vi "Motor PWM.vi"() -> ()   [LabVIEW 2018]
panel:
  in  "Nome do canal":tag="C/PWM0"
  in  "stop":bool
  in  "PWM freq [Hz]":dbl(slide)=100.0 scale=40.0..40000.0
  in  "PWM duty  [%]":dbl(slide) scale=0.0..100.0
  in  "Iniciar o controle":bool
  # "CONTROLE DO MOTOR COM SINAL DE PWM"
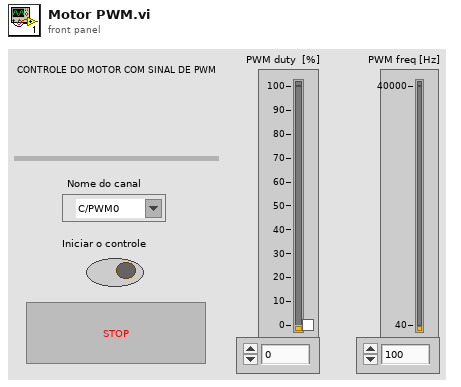
[diagram p1: front panel]
types:
  T1 = typedef "PWM.lvlib/PWM Reference.ctl" = cluster{"myRIO Reference":T2, "PWM Channels Enum":T6, "PWM Configuration":T7}
  T2 = typedef "myRIO Generic Hardware Reference.ctl" = cluster{"myRIO Model":T3, "myRIO Hardware Reference":T4}
  T3 = typedef "Hardware Version Enum.ctl" = enum16{"Unknown", "myRIO-1900", "myRIO-1950", "roboRIO", "NI ELVIS RIO CM"}
  T4 = typedef "myRIO v1.0 Reference.ctl" = cluster{"Generic FPGA Reference":T5, "Allow multiple opens":bool}
  T5 = typedef "Generic FPGA Reference.ctl" = refnum<k20>
  T6 = typedef "PWM Channels Enum.ctl" = enum16{"Not Connected", "C/PWM0", "C/PWM1", "A/PWM0", "A/PWM1", "A/PWM2", "B/PWM0", "B/PWM1", "B/PWM2", "PWM/PWM0", "PWM/PWM1", "PWM/PWM2", "PWM/PWM3", "PWM/PWM4", "PWM/PWM5", "PWM/PWM6", "PWM/PWM7", "PWM/PWM8", "PWM/PWM9"}
  T7 = typedef "PWM.lvlib/PWM Configuration.ctl" = cluster{"Frequency":dbl, "Duty Cycle":dbl}
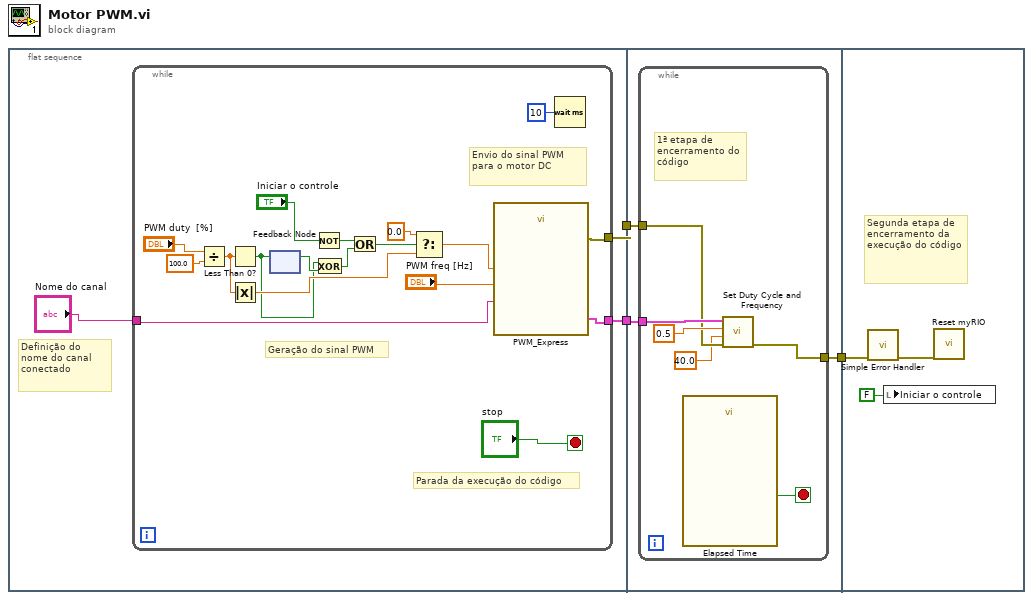
[diagram p0: block diagram]
diagram:
  n1 = flat-sequence {
    tunnel: [w6] -> w3
    tunnel: [w4] -> w2
    tunnel: w3 -> [w26]
    tunnel: w2 -> [w27]
    tunnel: [w25] -> w1
    tunnel: w1 -> [w34]
    frame #0 {
      # "Definição do nome do canal conectado"
      n2 = while {
        tunnel: [w13] -> w6
        tunnel: "Nome do canal" -> [w8]
        tunnel: [w7] -> w4
        stop <- "stop" stop-if-true
        # "Parada da execução do código"
        # "Envio do sinal PWM para o motor DC"
        # "Geração do sinal PWM"
        n3 = Divide(x="PWM duty  [%]", y=100.0) -> (x/y=w17:dbl)
        n4 = Less Than 0?(x=w17) -> (x < 0?=w14:bool)
        n5 = Absolute Value(x=w17) -> (abs(x)=w16:dbl)
        n6 = feedback #1() -> (w23:bool)  [unwired: 1 in]
        n7 = feedback-in #1(w14) -> ()
        n8 = Not(x="Iniciar o controle") -> (.not. x?=w19:bool)
        n9 = Exclusive Or(1:w23, 2:w14) -> (0:w21:bool)
        n10 = Or(x=w19, y=w21) -> (x .or. y?=w20:bool)
        n11 = Select(t=0.0 ("f"), s=w20, f=w16) -> (s? t:f=w9:dbl)
        n12 = call "PWM_Express.vi"("Channel Name"=w8, "Frequency [Hz]"="PWM freq [Hz]", "Duty Cycle"=w9) -> ("error out"=w13:errorcluster, "PWM Ref Out"=w7:T1)  [unwired: 3 in]
        n13 = Wait (ms)(milliseconds to wait=u32 10) -> ()  [unwired: 1 out]
      }
    }
    frame #1 {
      n14 = while {
        tunnel: w27 -> [w33]
        tunnel: w26 -> [w31]
        tunnel: [w28] -> w25
        stop <- w30 stop-if-true
        # "1ª etapa de encerramento do código"
        n15 = call "Elapsed Time"() -> ("Time has Elapsed"=w30:bool)  [unwired: 12 in, 7 out]
        n16 = call <vilib>:"Set Duty Cycle and Frequency.vi"("error in (no error)"=w31, "Frequency [Hz]"=40.0, "Duty Cycle"=0.5, "PWM Ref In"=w33) -> ("error out"=w28:errorcluster)  [unwired: 5 in, 1 out]
      }
    }
    frame #2 {
      # "Segunda etapa de encerramento da execução do código"
      n17 = call <vilib>:"Simple Error Handler.vi"("error in (no error)"=w34) -> ("error out"=w36:errorcluster)  [unwired: 4 in, 4 out]
      n18 = local write "Iniciar o controle"(FALSE) -> ()
      n19 = call <vilib>:"Reset myRIO.vi"("error in (no error)"=w36) -> ()  [unwired: 10 in, 1 out]
    }
  }
